vi "time_step.vi"(0 "Iterations per time step":i32, 1 "Microwave on":bool=TRUE, 5 "Time step (s)":dbl, 7 "Internal parameters in":T4, 9 "System parameters":T2, 11 "Physical constants":T3, 12 "Fit parameters":T1) -> (8 "Internal parameters out":T4)   [LabVIEW 2015]
uses:
  Simulation (old)/internal_parameters.ctl
  Simulation (old)/physical_constants.ctl
  Simulation (old)/system_parameters.ctl
  Simulation (old)/fit_parameters.ctl
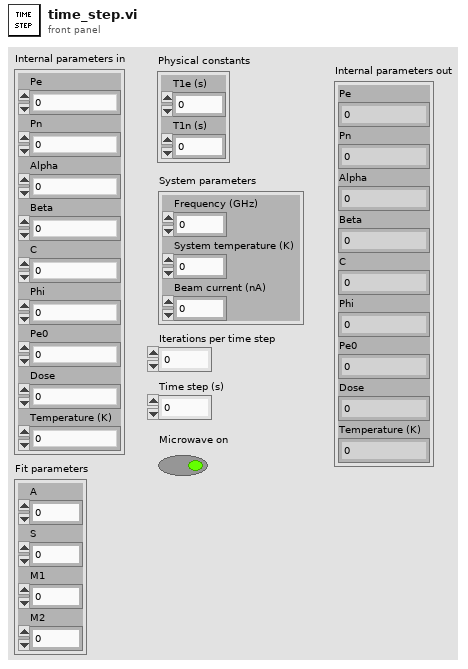
[diagram p1: front panel]
types:
  T1 = typedef "fit_parameters.ctl" = cluster{"A":dbl, "S":dbl, "M1":dbl, "M2":dbl}
  T2 = typedef "system_parameters.ctl" = cluster{"Frequency (GHz)":dbl, "System temperature (K)":dbl, "Beam current (nA)":dbl}
  T3 = typedef "physical_constants.ctl" = cluster{"T1e (s)":dbl, "T1n (s)":dbl}
  T4 = typedef "internal_parameters.ctl" = cluster{"Pe":dbl, "Pn":dbl, "Alpha":dbl, "Beta":dbl, "C":dbl, "Phi":dbl, "Pe0":dbl, "Dose":dbl, "Temperature (K)":dbl}
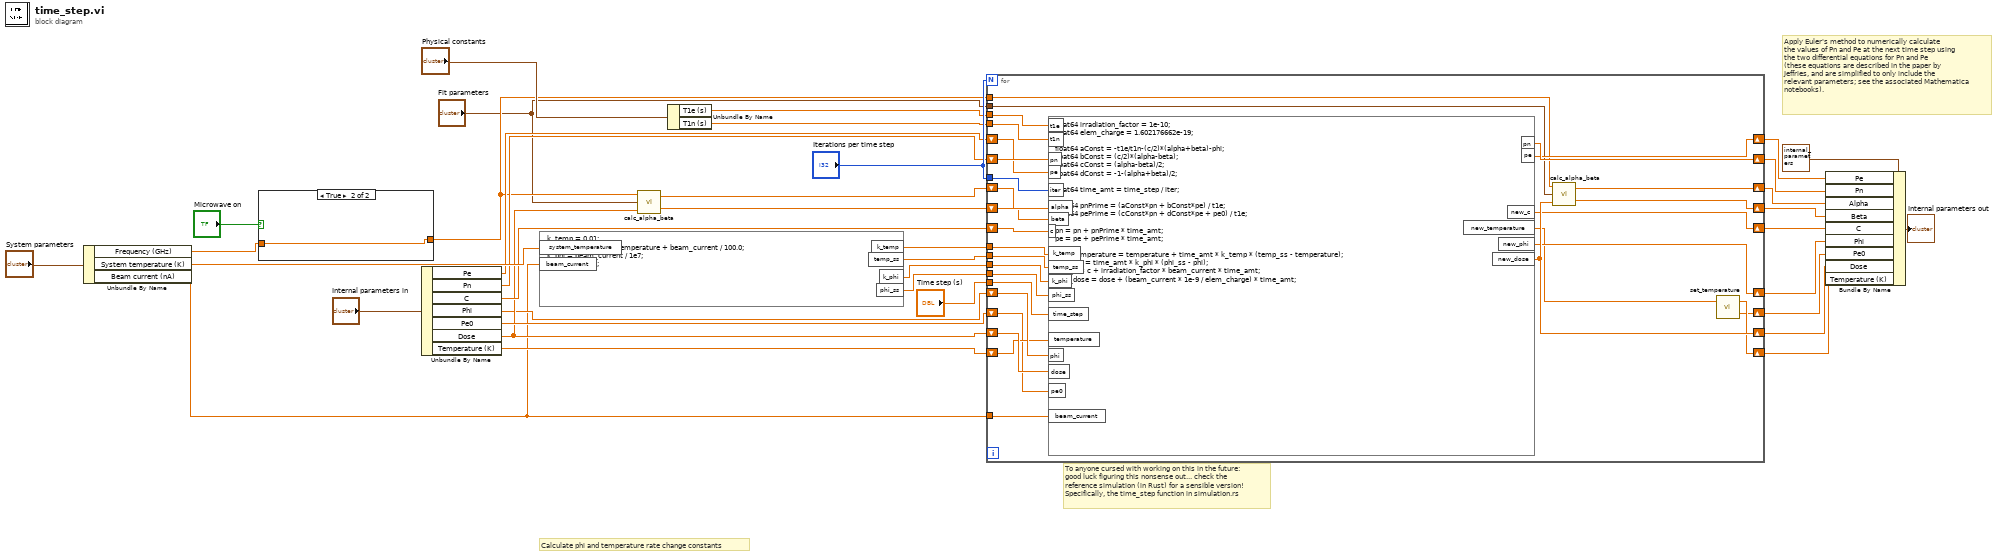
[diagram p0: block diagram]
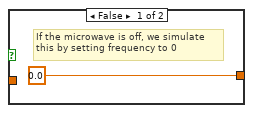
[diagram p2: hidden frame]
diagram:
  # "To anyone cursed with working on this in the future:\ngood luck figuring this nonsense out... check the\nreference simulation (in Rust) for a sensible version!\nSpecifically, the time_step function in simulation.rs"
  # "Apply Euler's method to numerically calculate\nthe values of Pn and Pe at the next time step using\nthe two differential equations for Pn and Pe\n(these equations are described in the paper by\nJeffries, and are simplified to only include the\nrelevant parameters; see the associated Mathematica\nnotebooks)."
  # "Calculate phi and temperature rate change constants"
  n1 = Unbundle By Name("System parameters") -> ("Frequency (GHz)"=w3:dbl, "System temperature (K)"=w26:dbl, "Beam current (nA)"=w16:dbl)
  n2 = case shown="True" "Microwave on" {
    tunnel: w3 -> [_ w39]
    tunnel: [0.0 ("Frequency") w39] -> w2
    frame False {
      # "If the microwave is off, we simulate\nthis by setting frequency to 0"
    }
    frame True {
    }
  }
  n3 = Unbundle By Name("Internal parameters in") -> ("Pe"=w23:dbl, "Pn"=w22:dbl, "C"=w21:dbl, "Phi"=w18:dbl, "Pe0"=w20:dbl, "Dose"=w19:dbl, "Temperature (K)"=w17:dbl)
  n4 = formula code="k_temp = 0.01;\ntemp_ss = system_temperature + beam_current / 100.0;\nk_phi = beam_current / 1e7;\nphi_ss = 0.001;"("system_temperature"=w26, "beam_current"=w16) -> ("k_temp"=w37:dbl, "temp_ss"=w36:dbl, "k_phi"=w35:dbl, "phi_ss"=w34:dbl)
  n5 = call "calc_alpha_beta.vi"("Dose"=w19, "Fit parameters"="Fit parameters", "Frequency (GHz)"=w2) -> ("Beta"=w32:dbl, "Alpha"=w33:dbl)
  n6 = Unbundle By Name("Physical constants") -> ("T1e (s)"=w25:dbl, "T1n (s)"=w24:dbl)
  n7 = for {
    N: "Iterations per time step" -> [_]
    shift-right: [w67] -> w6
    shift-left: w22 -> [w69]
    shift-right: [w66] -> w5
    shift-left: w23 -> [w68]
    tunnel: w37 -> [w65]
    tunnel: w36 -> [w64]
    tunnel: w35 -> [w63]
    tunnel: w34 -> [w62]
    tunnel: "Time step (s)" -> [w61]
    shift-right: [w56] -> w8
    shift-left: w33 -> [w60]
    shift-right: [w55] -> w7
    shift-left: w32 -> [w59]
    shift-right: [w50] -> w9
    shift-left: w21 -> [w58]
    shift-right: [w54] -> w12
    shift-left: w19 -> [w57]
    shift-right: [w52] -> w10
    shift-left: w18 -> [w53]
    shift-right: [w48] -> w13
    shift-left: w17 -> [w51]
    shift-right: [w46] -> w11
    shift-left: w20 -> [w49]
    tunnel: "Iterations per time step" -> [w45]
    tunnel: w2 -> [w44]
    tunnel: w25 -> [w43]
    tunnel: w24 -> [w42]
    tunnel: w16 -> [w41]
    tunnel: "Fit parameters" -> [w40]
    n8 = formula code="float64 irradiation_factor = 1e-10;\nfloat64 elem_charge = 1.602176662e-19;\n\nfloat64 aConst = -t1e/t1n-(c/2)*(alpha+beta)-phi;\nfloat64 bConst = (c/2)*(alpha-beta);\nfloat64 cConst = (alpha-beta)/2;\nfloat64 dConst = -1-(alpha+beta)/2;\n\nfloat64 time_amt = time_step / iter;\n\nfloat64 pnPrime = (aConst*pn + bConst*pe) / t1e;\nfloat64 pePrime = (cConst*pn + dConst*pe + pe0) / t1e;\n\npn = pn + pnPrime * time_amt;\npe = pe + pePrime * time_amt;\n\nnew_temperature = temperature + time_amt * k_temp * (temp_ss - temperature);\nnew_phi = time_amt * k_phi * (phi_ss - phi);\nnew_c = c + irradiation_factor * beam_current * time_amt;\nnew_dose = dose + (beam_current * 1e-9 / elem_charge) * time_amt;"("pn"=w69, "pe"=w68, "t1e"=w43, "iter"=w45, "alpha"=w60, "beta"=w59, "c"=w58, "t1n"=w42, "k_temp"=w65, "temp_ss"=w64, "k_phi"=w63, "phi_ss"=w62, "temperature"=w51, "time_step"=w61, "phi"=w53, "dose"=w57, "pe0"=w49, "beam_current"=w41) -> ("pn"=w67:dbl, "pe"=w66:dbl, "new_temperature"=w47:dbl, "new_phi"=w52:dbl, "new_dose"=w54:dbl, "new_c"=w50:dbl)
    n9 = call "calc_alpha_beta.vi"("Dose"=w54, "Fit parameters"=w40, "Frequency (GHz)"=w44) -> ("Beta"=w55:dbl, "Alpha"=w56:dbl)
    n10 = call "set_temperature.vi"("Temperature in"=w47) -> ("Pe0 out"=w46:dbl, "Temperature out"=w48:dbl)  [unwired: 1 in]
  }
  n11 = Bundle By Name(cluster=T4 {"Pe"=0.0, "Pn"=0.0, "Alpha"=0.0, "Beta"=0.0, "C"=0.0, "Phi"=0.0, "Pe0"=0.0, "Dose"=0.0, "Temperature (K)"=0.0} ("Simulation parameters out"), "Pe"=w5, "Pn"=w6, "Alpha"=w8, "Beta"=w7, "C"=w9, "Phi"=w10, "Pe0"=w11, "Dose"=w12, "Temperature (K)"=w13) -> (→"Internal parameters out":T4)
